vi "Agilent DMM Acutal Range.vi"(9 "Coerced Range":T1, 10 "Available Ranges":T1[](array[typedef])) -> (1 "Acutal Range":T1)   [LabVIEW 2011]
uses:
  TypeDefs/Agilent DMM Range.ctl
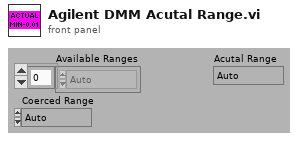
[diagram p1: front panel]
types:
  T1 = typedef "Agilent DMM Range.ctl" = enum16{"Auto", "Min", "Max", "0.01", "0.1", "1", "3", "10", "100", "1,000", "10,000", "100,000", "1,000,000", "10,000,000", "100,000,000"}
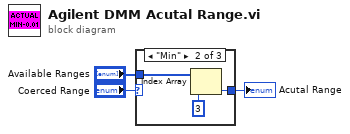
[diagram p0: block diagram]
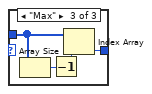
[diagram p3: hidden frame]
diagram:
  n1 = case shown="\"Min\"" "Coerced Range" {
    selector: "Coerced Range" -> [w4 _ _]
    tunnel: [w4 w6 w11] -> w1
    tunnel: "Available Ranges" -> [_ w7 w9]
    frame Default {
    }
    frame "Min" {
      n2 = Index Array(array=w7, index=3) -> (element=w6:T1)
    }
    frame "Max" {
      n3 = Array Size(array=w9) -> (size(s)=w10:i32)
      n4 = Decrement(x=w10) -> (x-1=w8:i32)
      n5 = Index Array(array=w9, index=w8) -> (element=w11:T1)
    }
  }
  "Acutal Range" <- w1
